vi "Endurance Set Operation.vi"(8 "error in (no error)":errorcluster, 9 "BLV":dbl=2.0 format="%#_13g", 10 "WLV":dbl=3.0 format="%#_13g", 11 "instrument handle":refnum<k15>="PXI1Slot2 (8)") -> (0 "error out":errorcluster, 3 "instrument handle out":refnum<k15>="PXI1Slot2 (8)")   [LabVIEW 2018]
uses:
  <instrlib>/niDigital/niDigital.llb/niDigital Burst Pattern (Burst Only).vi
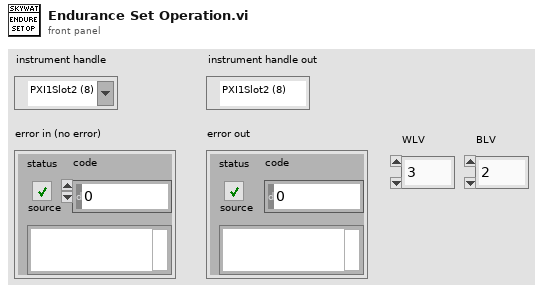
[diagram p1: front panel]
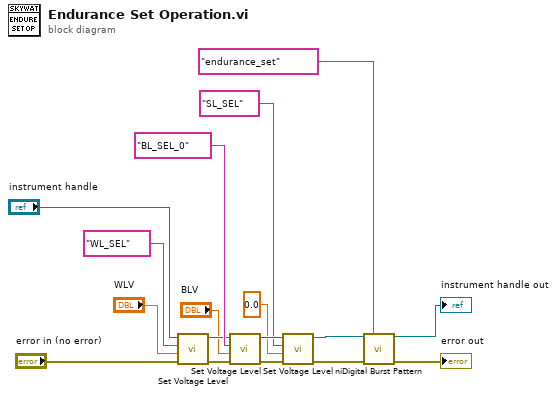
[diagram p0: block diagram]
diagram:
  n1 = call "Set Voltage Level.vi"("error in (no error)"="error in (no error)", "level (V)"="WLV", "channel list"="WL_SEL", "instrument handle"="instrument handle") -> ("error out"=w11:errorcluster, "instrument handle out"=w12:refnum<k15>)  [unwired: 6 in]
  n2 = call "Set Voltage Level.vi"("error in (no error)"=w11, "level (V)"="BLV", "channel list"="BL_SEL_0", "instrument handle"=w12) -> ("error out"=w10:errorcluster, "instrument handle out"=w13:refnum<k15>)  [unwired: 6 in]
  n3 = call "Set Voltage Level.vi"("error in (no error)"=w10, "level (V)"=0.0, "channel list"="SL_SEL", "instrument handle"=w13) -> ("error out"=w5:errorcluster, "instrument handle out"=w7:refnum<k15>)  [unwired: 6 in]
  n4 = call-poly <instrlib>:"niDigital Burst Pattern.vi"("instrument handle"=w7, "start label"="endurance_set", "error in"=w5) -> ("instrument handle out"=→"instrument handle out":refnum<k15>, "error out"=→"error out":errorcluster)  [unwired: 11 in]
